vi "key.vi"() -> ()   [LabVIEW 2014]
panel:
  in  "Key":enum16{"Right", "Left", "Up", "Down"}(ring)
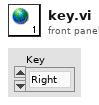
[diagram p1: front panel]
diagram:
